vi "ArmBegin.vi"(8 "error in (no error)":errorcluster) -> (0 "error out":errorcluster)   [LabVIEW 2020]
doc: "Begin for Arm\n\nInputs:\n -- Error in -- Error cluster -- propagated error input\n--DegreesInCircle--Double--\n--RevolutionsCountPerRotation--Double--\n\nOutputs:\n -- Error out -- Error cluster -- progated error output"
uses:
  <vilib>/Rock Robotics/WPI/Solenoid/WPI_SolenoidChannel.ctl
  <vilib>/Rock Robotics/WPI/ThirdParty/REV Robotics/REVLib/Typedef/Spark MAX Idle Mode.ctl
  <vilib>/Rock Robotics/WPI/ThirdParty/REV Robotics/REVLib/Typedef/Spark MAX Motor Type.ctl
  <vilib>/Rock Robotics/WPI/ThirdParty/Phoenix-LabVIEW/Motor Controller/Controls/CTRE_Phoenix_MotorControl_NeutralMode.ctl
  <vilib>/Rock Robotics/WPI/Encoder/WPI_EncoderType.ctl
  <vilib>/Rock Robotics/SystemInterfaces/DIO/FPGA_DIOChannel.ctl
  <vilib>/Rock Robotics/WPI/Solenoid/WPI_SolenoidOpenSingle.vi
  <vilib>/Rock Robotics/WPI/Counter/WPI_CounterDigitalInputToDigitalSource.vi
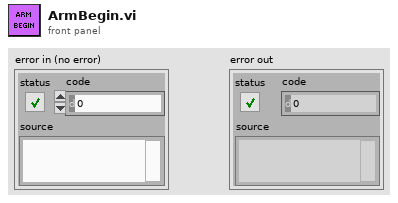
[diagram p1: front panel]
types:
  T1 = typedef "WPI_SolenoidChannel.ctl" = enum8{"Solenoid 0", "Solenoid 1", "Solenoid 2", "Solenoid 3", "Solenoid 4", "Solenoid 5", "Solenoid 6", "Solenoid 7", "Solenoid 8", "Solenoid 9", "Solenoid 10", "Solenoid 11", "Solenoid 12", "Solenoid 13", "Solenoid 14", "Solenoid 15", "Invalid"}
  T2 = typedef "Spark MAX Idle Mode.ctl" = enum16{"Coast", "Brake"}
  T3 = typedef "Spark MAX Motor Type.ctl" = enum16{"Brushed", "Brushless"}
  T4 = typedef "CTRE_Phoenix_MotorControl_NeutralMode.ctl" = enum8{"EEPROMSetting", "Override to Coast", "Override to Brake"}
  T5 = typedef "WPI_EncoderType.ctl" = enum16{"1x", "2x", "4x"}
  T6 = typedef "FPGA_DIOChannel.ctl" = enum8{"DIO 0", "DIO 1", "DIO 2", "DIO 3", "DIO 4", "DIO 5", "DIO 6", "DIO 7", "DIO 8", "DIO 9", "DIO MXP 0", "DIO MXP 1", "DIO MXP 2", "DIO MXP 3", "DIO MXP 4", "DIO MXP 5", "DIO MXP 6", "DIO MXP 7", "DIO MXP 8", "DIO MXP 9", "DIO MXP 10", "DIO MXP 11", "DIO MXP 12", "DIO MXP 13", "DIO MXP 14", "DIO MXP 15", "SPI Port CS1", "SPI Port CS2", "SPI Port CS3", "SPI Port MISO", "SPI Port MOSI", "Invalid"}
  T7 = typedef "WPI_MotorControlDeviceRef.ctl" = cluster{"DeviceStatus":errorcluster, "Type":T8, "PWM":cluster{"PWM Channel":T9, "DeadBand":T10}, "CAN":cluster{"Device Number":u8, "SetOutput VI Ref":variant, "GetOutput VI Ref":variant, "Enable VI Ref":variant, "Disable VI Ref":variant, "Data":variant}, "Invert":bool, "DIO PWM":cluster{"PWM \"Enable\" Channel":T9, "DIOChannel":T6, "PWM Rate":dbl}}
  T8 = typedef "WPI_MotorControlType.ctl" = enum16{"PWM", "CAN", "DIO PWM"}
  T9 = typedef "FPGA_DIOPWMChannel.ctl" = enum8{"PWM 0", "PWM 1", "PWM 2", "PWM 3", "PWM 4", "PWM 5", "PWM 6", "PWM 7", "PWM 8", "PWM 9", "PWM MXP 0", "PWM MXP 1", "PWM MXP 2", "PWM MXP 3", "PWM MXP 4", "PWM MXP 5", "PWM MXP 6", "PWM MXP 7", "PWM MXP 8", "PWM MXP 9", "Invalid"}
  T10 = typedef "WPI_PWMDeadband.ctl" = cluster{"Name":string, "maxPositivePwm":i32, "minPositivePwm":i32, "centerPwm":i32, "maxNegativePwm":i32, "minNegativePwm":i32, "angularRange":u16}
  T11 = typedef "WPI_SolenoidDevRef.ctl" = cluster{"DevStatus":errorcluster, "Pneumatics Control Module":u8, "Forward Solenoid Channel":T1, "Reverse Solenoid Channel":T1}
  T12 = typedef "WPI_DigitalInputDevRef.ctl" = cluster{"DevStatus":errorcluster, "DIO Channel":T6}
  T13 = typedef "FPGA_CounterEncoderSourceConvertionLVSourceType.ctl" = cluster{"DevStatus":errorcluster, "AnalogTriggerMode?":bool, "DigitalMode":cluster{"DIO Channel":T14}, "AnalogTriggerMode":cluster{"AnalogTriggerIndex":T15, "OutputType":T16}}
  T14 = typedef "FPGA_DIODigitalSourceChannel.ctl" = enum8{"DIO 0", "DIO 1", "DIO 2", "DIO 3", "DIO 4", "DIO 5", "DIO 6", "DIO 7", "DIO 8", "DIO 9", "DIO MXP 0", "DIO MXP 1", "DIO MXP 2", "DIO MXP 3", "DIO MXP 4", "DIO MXP 5", "DIO MXP 6", "DIO MXP 7", "DIO MXP 8", "DIO MXP 9", "DIO MXP 10", "DIO MXP 11", "DIO MXP 12", "DIO MXP 13", "DIO MXP 14", "DIO MXP 15", "SPI Port CS1", "SPI Port CS2", "SPI Port CS3", "SPI Port MISO", "SPI Port MOSI", "Disabled"}
  T15 = typedef "FPGA_AnalogTriggerIndex.ctl" = enum8{"Trig 0", "Trig 1", "Trig 2", "Trig 3", "Trig 4", "Trig 5", "Trig 6", "Trig 7", "Invalid"}
  T16 = typedef "FPGA_AnalogTriggerOutType.ctl" = enum16{"InWindow", "TriggerState", "Rising", "Falling"}
  T17 = typedef "WPI_EncoderDevRef.ctl" = cluster{"DevStatus":errorcluster, "EncoderIndex":T18, "CounterIndex":T19, "DistancePerCount":dbl, "Decoding Type":T5}
  T18 = typedef "FPGA_EncoderIdx.ctl" = enum8{"Enc 0", "Enc 1", "Enc 2", "Enc 3", "Enc 4", "Enc 5", "Enc 6", "Enc 7", "Invalid"}
  T19 = typedef "FPGA_CounterCtrSystemIndex.ctl" = enum8{"Ctr 0", "Ctr 1", "Ctr 2", "Ctr 3", "Ctr 4", "Ctr 5", "Ctr 6", "Ctr 7", "Invalid"}
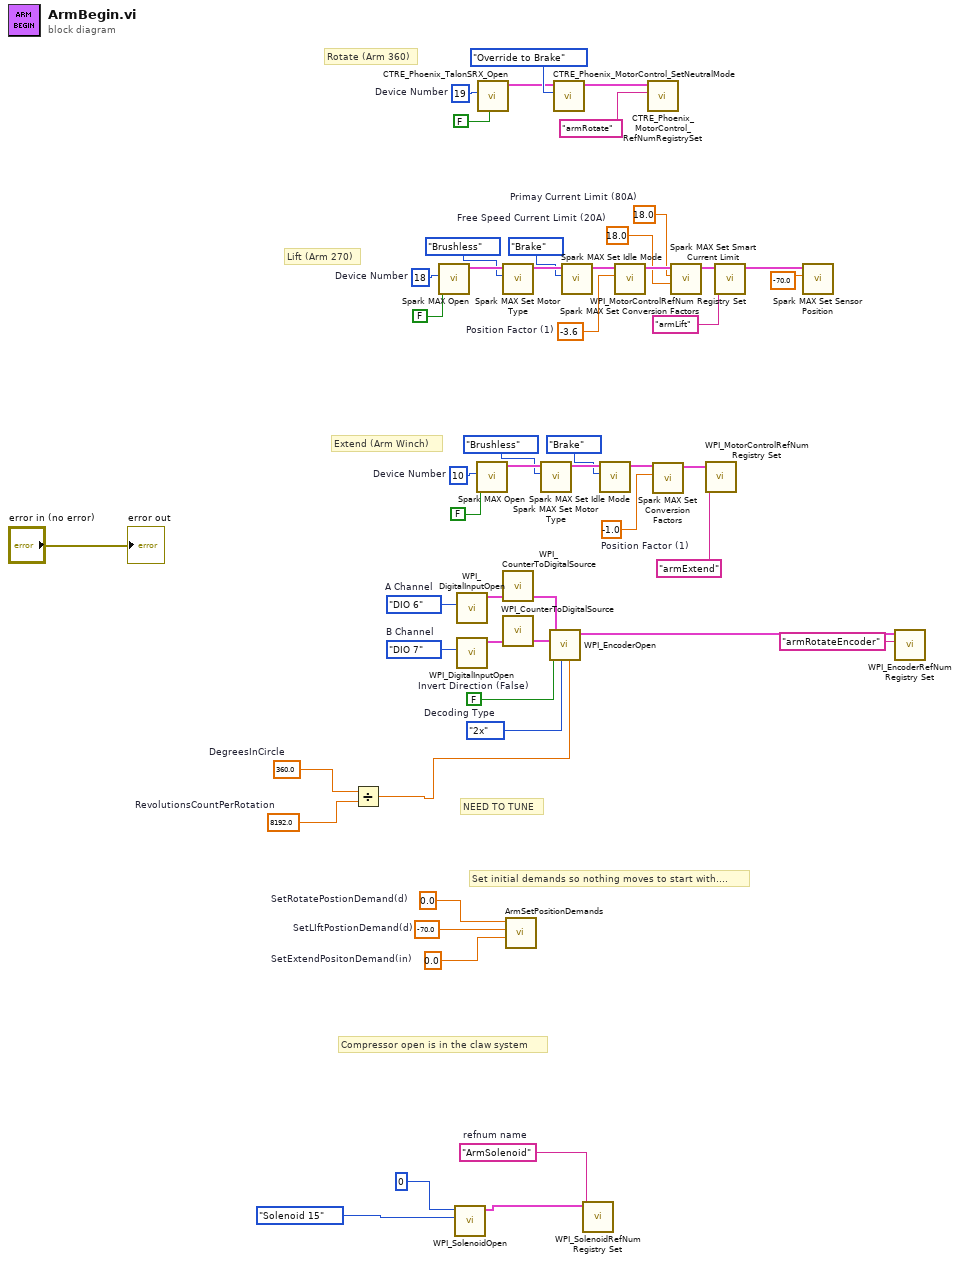
[diagram p0: block diagram]
diagram:
  w3 = 0.0  # SetRotatePostionDemand(d)
  w4 = -70.0  # SetLIftPostionDemand(d)
  w5 = 0.0  # SetExtendPositonDemand(in)
  w6 = "ArmSolenoid"  # refnum name
  w10 = 18.0  # Free Speed Current Limit (20A)
  w11 = 18.0  # Primay Current Limit (80A)
  w15 = 8192.0  # RevolutionsCountPerRotation
  w16 = 360.0  # DegreesInCircle
  w23 = -3.6  # Position Factor (1)
  w30 = u8 18  # Device Number
  w33 = -1.0  # Position Factor (1)
  w40 = u8 10  # Device Number
  w20 = u8 19  # Device Number
  w44 = FALSE  # Invert Direction (False)
  w45 = WPI_EncoderType."2x"  # Decoding Type
  w49 = FPGA_DIOChannel."DIO 7"  # B Channel
  w48 = FPGA_DIOChannel."DIO 6"  # A Channel
  # "Set initial demands so nothing moves to start with...."
  # "Compressor open is in the claw system"
  # "NEED TO TUNE"
  # "Lift (Arm 270)"
  # "Extend (Arm Winch)"
  # "Rotate (Arm 360)"
  n1 = Divide(x=w16, y=w15) -> (x/y=w14:dbl)
  n2 = call <vilib>:"Spark MAX Open.vi"("Invert"=FALSE, "Device Number"=w30) -> ("MotorControlDeviceRef"=w28:T7)  [unwired: 8 in, 1 out]
  n3 = call-poly <vilib>:"WPI_SolenoidOpen.vi"("Solenoid Channel"=WPI_SolenoidChannel."Solenoid 15" ("Forward Solenoid Channel"), "Pneumatics Device (def)"=u8 0) -> ("SolenoidDevRef"=w7:T11)  [unwired: 8 in, 1 out]
  n4 = call <vilib>:"WPI_DigitalInputOpen.vi"("DIO Channel"=w48) -> ("DigitalInputDevRef"=w46:T12)  [unwired: 1 in, 9 out]
  n5 = call <vilib>:"WPI_DigitalInputOpen.vi"("DIO Channel"=w49) -> ("DigitalInputDevRef"=w47:T12)  [unwired: 1 in, 9 out]
  n6 = call <vilib>:"Spark MAX Open.vi"("Invert"=FALSE, "Device Number"=w40) -> ("MotorControlDeviceRef"=w38:T7)  [unwired: 8 in, 1 out]
  n7 = call <vilib>:"CTRE_Phoenix_TalonSRX_Open.vi"("Invert"=FALSE, "Device Number"=w20) -> ("PhoenixMotorControlDevRef"=w21:T7)  [unwired: 8 in, 1 out]
  n8 = call <vilib>:"Spark MAX Set Motor Type.vi"("Motor Type"=Spark_MAX_Motor_Type."Brushless", "MotorControlDevRef"=w28) -> ("MotorControlDeviceRef"=w27:T7)  [unwired: 8 in, 1 out]
  n9 = call-poly <vilib>:"WPI_CounterToDigitalSource.vi"("DigitalInputDevRef"=w46) -> ("Digital Source"=w50:T13)  [unwired: 6 out]
  n10 = call-poly <vilib>:"WPI_CounterToDigitalSource.vi"("DigitalInputDevRef"=w47) -> ("Digital Source"=w51:T13)  [unwired: 6 out]
  n11 = call "ArmSetPositionDemands.vi"("SetExtendPositonDemand(in)"=w5, "SetLIftPostionDemand(d)"=w4, "SetRotatePostionDemand(d)"=w3) -> ()  [unwired: 9 in]
  n12 = call <vilib>:"Spark MAX Set Motor Type.vi"("Motor Type"=Spark_MAX_Motor_Type."Brushless", "MotorControlDevRef"=w38) -> ("MotorControlDeviceRef"=w37:T7)  [unwired: 8 in, 1 out]
  n13 = call <vilib>:"WPI_EncoderOpen.vi"("DistancePerCount"=w14, "Decoding Type"=w45, "Invert Direction (False)"=w44, "BSource"=w51, "ASource"=w50) -> ("EncoderDevRef"=w43:T17)  [unwired: 5 in, 1 out]
  n14 = call <vilib>:"CTRE_Phoenix_MotorControl_SetNeutralMode.vi"("Motor Control Neutral Mode"=CTRE_Phoenix_MotorControl_NeutralMode."Override to Brake", "PhoenixMotorControlDevRef"=w21) -> ("PhoenixMotorControlDevRef"=w18:T7)  [unwired: 8 in, 1 out]
  n15 = call <vilib>:"Spark MAX Set Idle Mode.vi"("Idle Mode"=Spark_MAX_Idle_Mode."Brake", "MotorControlDeviceRef in"=w27) -> ("MotorControlDeviceRef out"=w24:T7)  [unwired: 8 in, 1 out]
  n16 = call <vilib>:"WPI_SolenoidRefNum Registry Set.vi"("refnum name"=w6, "SolenoidDevRef"=w7) -> ()  [unwired: 8 in, 2 out]
  n17 = call <vilib>:"Spark MAX Set Idle Mode.vi"("Idle Mode"=Spark_MAX_Idle_Mode."Brake", "MotorControlDeviceRef in"=w37) -> ("MotorControlDeviceRef out"=w34:T7)  [unwired: 8 in, 1 out]
  n18 = call <vilib>:"Spark MAX Set Conversion Factors.vi"("Position Factor (1)"=w23, "MotorControlDeviceRef in"=w24) -> ("MotorControlDeviceRef out"=w13:T7)  [unwired: 8 in, 1 out]
  n19 = call <vilib>:"CTRE_Phoenix_MotorControl_RefNumRegistrySet.vi"("refnum name"="armRotate", "PhoenixMotorControlDevRef"=w18) -> ()  [unwired: 8 in, 2 out]
  n20 = call <vilib>:"Spark MAX Set Conversion Factors.vi"("Position Factor (1)"=w33, "MotorControlDeviceRef in"=w34) -> ("MotorControlDeviceRef out"=w32:T7)  [unwired: 8 in, 1 out]
  n21 = call <vilib>:"Spark MAX Set Smart Current Limit.vi"("Free Speed Current Limit (20A)"=w10, "Primay Current Limit (80A)"=w11, "MotorControlDeviceRef in"=w13) -> ("MotorControlDeviceRef out"=w12:T7)  [unwired: 7 in, 1 out]
  n22 = call <vilib>:"WPI_MotorControlRefNum Registry Set.vi"("refnum name"="armExtend", "MotorControlDevRef"=w32) -> ()  [unwired: 8 in, 2 out]
  n23 = call <vilib>:"WPI_MotorControlRefNum Registry Set.vi"("refnum name"="armLift", "MotorControlDevRef"=w12) -> ("MotorControlDevRef"=w2:T7)  [unwired: 8 in, 1 out]
  n24 = call <vilib>:"Spark MAX Set Sensor Position.vi"("Position"=-70.0, "MotorControlDeviceRef"=w2) -> ()  [unwired: 8 in, 2 out]
  n25 = call <vilib>:"WPI_EncoderRefNum Registry Set.vi"("refnum name"="armRotateEncoder", "EncoderDevRef"=w43) -> ()  [unwired: 8 in, 2 out]
  "error out" <- "error in (no error)"
